vi "Actor Core.vi"(8 "error in":errorcluster, 11 "File Dialog in":refnum<class "File Dialog.lvclass">) -> (0 "error out":errorcluster, 3 "Actor out":refnum<class "Actor.lvclass">)   [LabVIEW 2018, in "File Dialog Actor.lvlib" / "File Dialog.lvclass"]
doc: "(<B>Filename</B>: Actor Framework.lvlib:Actor.lvclass:Actor Core.vi)\n\nReceives messages to the actor, reacts to them, and initiates any error handling that may shut the actor down.\n\nDescendant classes may override this VI to append parallel tasks for the actor to complete while it handles messages. Overrides use the Call Parent Method node."
uses:
  File Dialog.lvclass
  C:/Program Files (x86)/National Instruments/LabVIEW 2018/vi.lib/ActorFramework/Actor/Actor.lvclass
  <vilib>/ActorFramework/Actor/Actor.lvclass
  <vilib>/ActorFramework/Actor/Actor.lvclass/Actor.ctl
  <vilib>/ActorFramework/Message Enqueuer/Message Enqueuer.lvclass/Message Enqueuer.ctl
  File Dialog.lvclass/File Dialog.ctl
  File Dialog Messages/Return File Path Msg/Return File Path Msg.lvclass/Return File Path Msg.ctl
  <vilib>/ActorFramework/Message Enqueuer/Init from Existing Queue.vi
  <vilib>/ActorFramework/Message Enqueuer/Enqueue.vi
  File Dialog Messages/Return File Path Msg/Return File Path Msg.lvclass
  C:/Program Files (x86)/National Instruments/LabVIEW 2018/vi.lib/ActorFramework/Message/Message.lvclass
  <vilib>/ActorFramework/Stop Msg/Stop Msg.lvclass
  <vilib>/ActorFramework/Message Priority Queue/Priority Enqueue.vi
  <vilib>/ActorFramework/Message Enqueuer/Message Enqueuer.lvclass
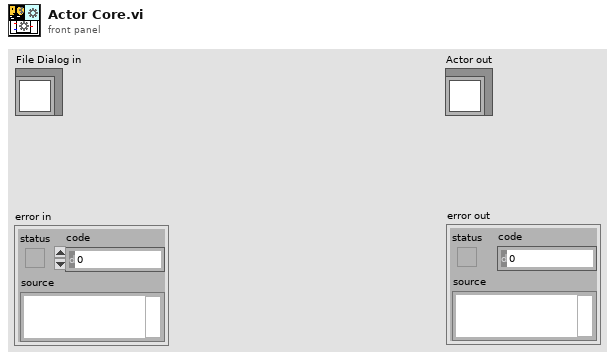
[diagram p1: front panel]
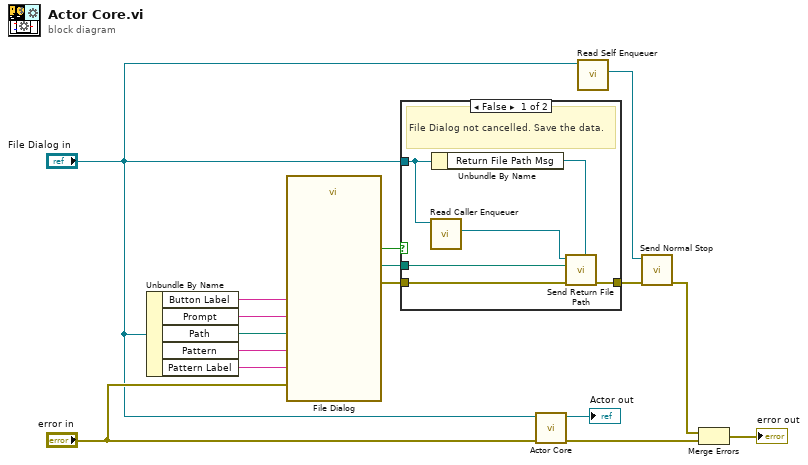
[diagram p0: block diagram]
diagram:
  n1 = Unbundle By Name("File Dialog in") -> ("Button Label"=w6:string, "Prompt"=w7:string, "Path"=w8:path, "Pattern"=w9:string, "Pattern Label"=w10:string)
  n2 = call "File Dialog"("start path"=w8, "prompt"=w7, "button label"=w6, "error in"="error in", "pattern (all files)"=w9, "pattern label"=w10) -> ("selected path"=w12:path, "cancelled"=w11:bool, "error out"=w13:errorcluster)  [unwired: 6 in, 1 out]
  n3 = case shown="False" w11 {
    tunnel: w12 -> [w19 _]
    tunnel: w13 -> [w20 w23]
    tunnel: "File Dialog in" -> [w22 _]
    tunnel: [w17 w23] -> w15
    frame False {
      # "File Dialog not cancelled. Save the data."
      n4 = call <vilib>:"Read Caller Enqueuer.vi"("Actor"=w22) -> ("Caller Enqueuer"=w21:refnum<class "Message Enqueuer.lvclass">)  [unwired: 10 in]
      n5 = Unbundle By Name(w22) -> ("Return File Path Msg"=w18:refnum<class "Return File Path Msg.lvclass">)
      n6 = call "Send Return File Path.vi"("Message Type"=w18, "error in"=w20, "File Path"=w19, "Message Enqueuer"=w21) -> ("error out"=w17:errorcluster)  [unwired: 6 in, 1 out]
    }
    frame True {
      # "Do nothing if the File Dialog was cancelled."
    }
  }
  n7 = call-parent "Actor Core.vi"("error in"="error in", "Actor in"="File Dialog in") -> ("error out"=w5:errorcluster, "Actor out"=→"Actor out":refnum<class "Actor.lvclass">)  [unwired: 8 in]
  n8 = call <vilib>:"Read Self Enqueuer.vi"("Actor"="File Dialog in") -> ("Self Enqueuer"=w16:refnum<class "Message Enqueuer.lvclass">)  [unwired: 10 in]
  n9 = call <vilib>:"Send Normal Stop.vi"("error in (no error)"=w15, "Message Enqueuer"=w16) -> ("error out"=w14:errorcluster)  [unwired: 9 in]
  n10 = Merge Errors(w14, w5) -> (→"error out":errorcluster)
